vi "Create (From VI Reference).vi"(8 "error in (no error)":errorcluster, 10 "VI":refnum<vi>) -> (0 "error out":errorcluster, 3 "JKI SM out":refnum<class "JKI SM.lvclass">)   [LabVIEW 2013, in "JKI State Machine API.lvlib" / "JKI SM.lvclass"]
uses:
  JKI SM.lvclass
  JKI SM.lvclass/JKI SM.ctl
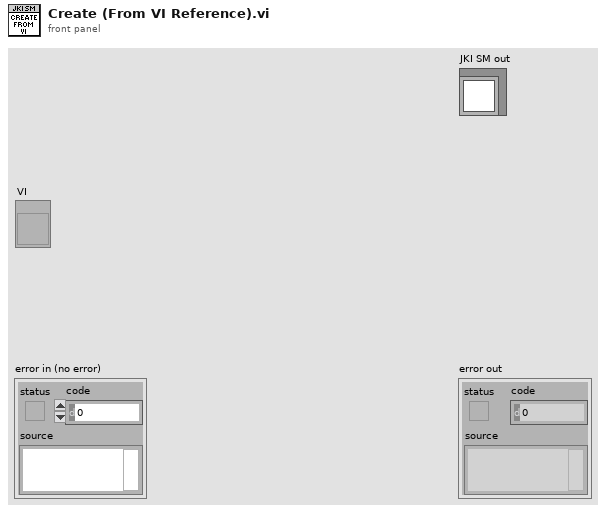
[diagram p1: front panel]
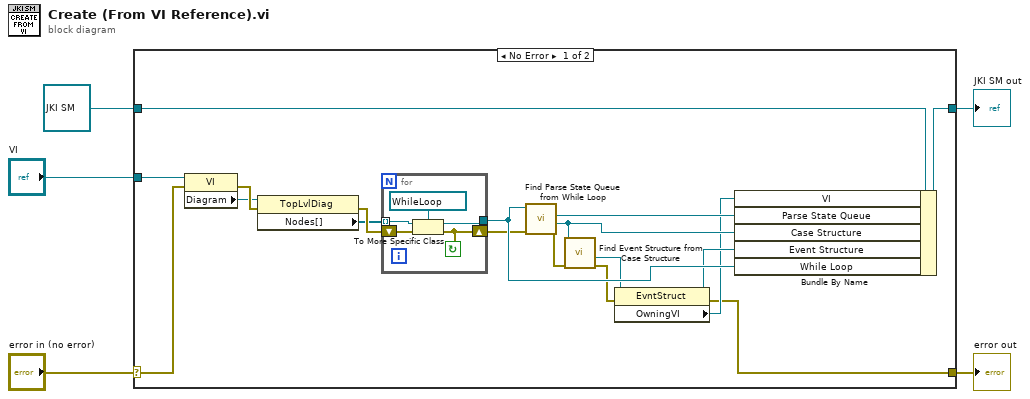
[diagram p0: block diagram]
diagram:
  n1 = case shown="No Error" "error in (no error)" {
    selector: "error in (no error)" -> [w18 w30]
    tunnel: [w6 w30] -> w4
    tunnel: [w16 w29] -> w2
    tunnel: refnum<class "JKI SM.lvclass"> refnum ("JKI SM") -> [w17 w29]
    tunnel: "VI" -> [w19 _]
    frame No Error {
      n2 = property class="VI"(reference=w19, error in=w18) -> (error out=w23:errorcluster, "Diagram"=w20:refnum<vi>)  [unwired: 1 out]
      n3 = property class="TopLvlDiag"(reference=w20, error in=w23) -> (error out=w22:errorcluster, "Nodes[]"=w21:refnum<vi>[])  [unwired: 1 out]
      n4 = for {
        tunnel: w21 -> [w27] mode=indexing
        tunnel: [w25] -> w13
        shift-right: [w24] -> w12
        shift-left: w22 -> [w26]
        stop <- w24 continue-if-true
        n5 = To More Specific Class(target class=refnum<vi> refnum ("WLoop Refnum"), reference=w27, error in=w26) -> (specific class reference=w25:refnum<vi>, error out=w24:errorcluster)
      }
      n6 = call "Find Parse State Queue from While Loop.vi"("error in (no error)"=w12, "WhileLoop in"=w13) -> ("error out"=w14:errorcluster, "CaseStructure"=w11:refnum<vi>, "Parse State Queue"=w15:refnum<vi>)  [unwired: 7 in]
      n7 = call "Find Event Structure from Case Structure.vi"("error in (no error)"=w14, "CaseStructure"=w11) -> ("error out"=w7:errorcluster, "EvntStruct Refnum"=w10:refnum<vi>)  [unwired: 8 in]
      n8 = property class="EvntStruct"(reference=w10, error in=w7) -> (reference out=w9:refnum<vi>, error out=w6:errorcluster, "OwningVI"=w8:refnum<vi>)
      n9 = Bundle By Name(cluster=w17, "VI"=w8, "Parse State Queue"=w15, "Case Structure"=w11, "Event Structure"=w9, "While Loop"=w13) -> (w16:refnum<class "JKI SM.lvclass">)
    }
    frame Error {
    }
  }
  "error out" <- w4
  "JKI SM out" <- w2
